vi "ELVIS III v1.0 Coerce AI Scaling.vi"(5 "Max Value":dbl[](array[numeric]), 7 "Min Value":dbl[](array[numeric]), 8 "error in (no error)":errorcluster, 10 "Channel List Size":i32) -> (0 "error out":errorcluster, 2 "Scale Constants Array":T1)   [LabVIEW 2021]
uses:
  <vilib>/myRIO/Common/Instrument Driver Framework/Utilities/typedefs/Analog Scaling Constants List.ctl
  <vilib>/myRIO/Common/Instrument Driver Framework/Utilities/typedefs/Analog Scaling Constants.ctl
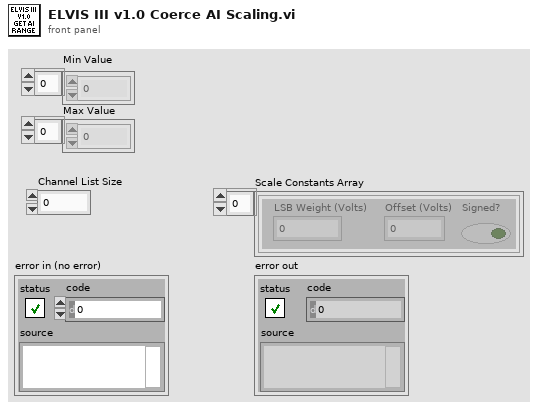
[diagram p1: front panel]
types:
  T1 = typedef "Analog Scaling Constants List.ctl" = T2[]
  T2 = typedef "Analog Scaling Constants.ctl" = cluster{"LSB Weight (Volts)":dbl, "Offset (Volts)":dbl, "Signed?":bool}
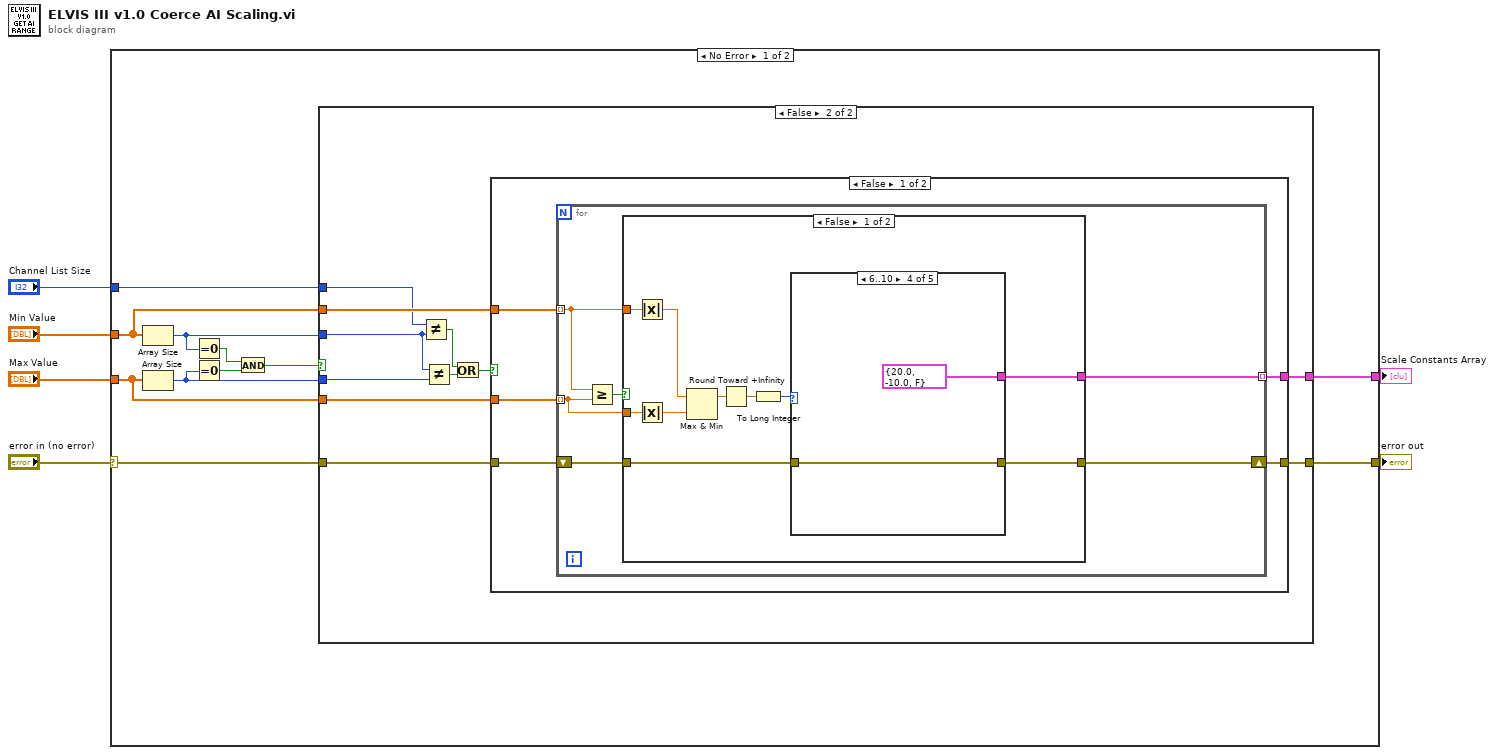
[diagram p0: block diagram]
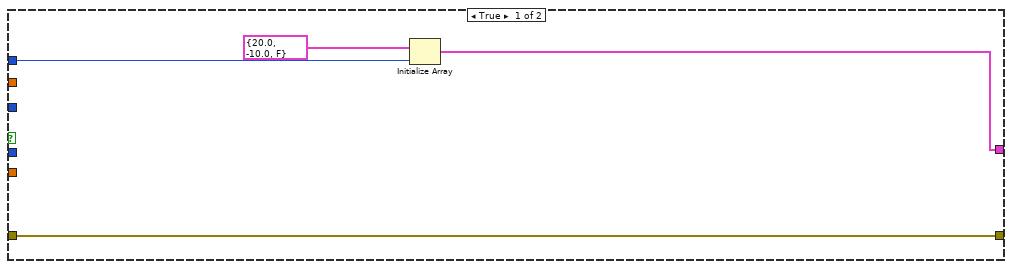
[diagram p2: hidden frame]
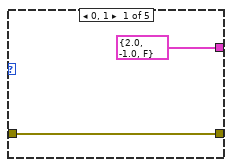
[diagram p3: hidden frame]
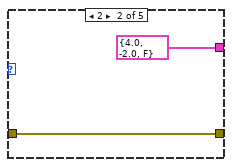
[diagram p4: hidden frame]
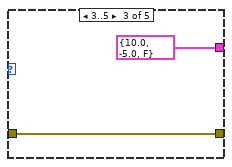
[diagram p5: hidden frame]
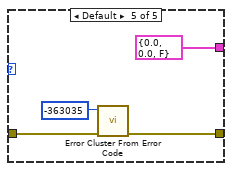
[diagram p6: hidden frame]
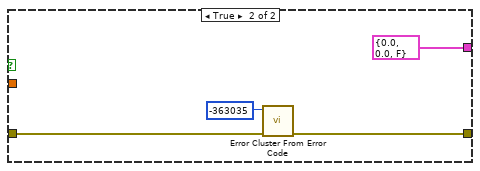
[diagram p7: hidden frame]
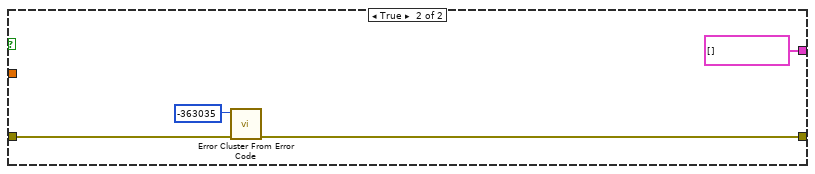
[diagram p8: hidden frame]
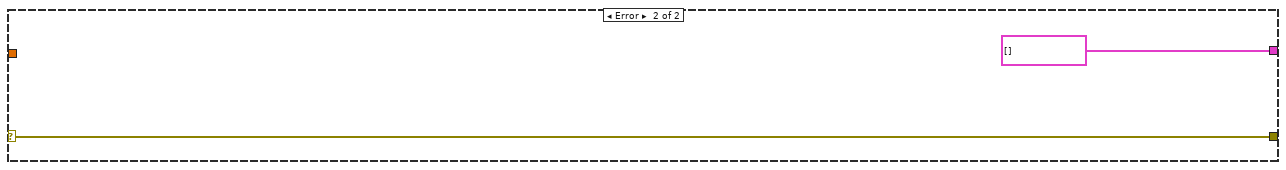
[diagram p9: hidden frame]
diagram:
  n1 = case shown="No Error" "error in (no error)" {
    selector: "error in (no error)" -> [w17 w75]
    tunnel: [w16 w75] -> w5
    tunnel: "Min Value" -> [w15 _]
    tunnel: "Max Value" -> [w14 _]
    tunnel: [w13 T2[] []] -> w2
    tunnel: "Channel List Size" -> [w12 _]
    frame No Error {
      n2 = Array Size(array=w15) -> (size(s)=w11:i32)
      n3 = Array Size(array=w14) -> (size(s)=w10:i32)
      n4 = Equal To 0?(x=w11) -> (x = 0?=w9:bool)
      n5 = Equal To 0?(x=w10) -> (x = 0?=w8:bool)
      n6 = And(x=w9, y=w8) -> (x .and. y?=w7:bool)
      n7 = case shown="False" w7 {
        tunnel: w17 -> [w21 w29]
        tunnel: [w21 w28] -> w16
        tunnel: w15 -> [_ w27]
        tunnel: w14 -> [_ w26]
        tunnel: [w18 w25] -> w13
        tunnel: w12 -> [w19 w24]
        tunnel: w11 -> [_ w23]
        tunnel: w10 -> [_ w22]
        frame True {
          n8 = Initialize Array(T2 {"LSB Weight (Volts)"=20.0, "Offset (Volts)"=-10.0, "Signed?"=FALSE} ("output cluster"), w19) -> (w18:T2[])
        }
        frame False {
          n9 = Not Equal?(x=w24, y=w23) -> (x != y?=w32:bool)
          n10 = Not Equal?(x=w23, y=w22) -> (x != y?=w31:bool)
          n11 = Or(x=w32, y=w31) -> (x .or. y?=w30:bool)
          n12 = case shown="False" w30 {
            tunnel: w29 -> [w35 w72]
            tunnel: [w34 w71] -> w28
            tunnel: w27 -> [w37 _]
            tunnel: w26 -> [w36 _]
            tunnel: [w33 T2[] []] -> w25
            frame False {
              n13 = for {
                tunnel: w37 -> [w40] mode=indexing
                tunnel: w36 -> [w39] mode=indexing
                shift-right: [w41] -> w34
                shift-left: w35 -> [w42]
                tunnel: [w38] -> w33 mode=indexing
                n14 = Greater Or Equal?(x=w40, y=w39) -> (x >= y?=w43:bool)
                n15 = case shown="False" w43 {
                  tunnel: w42 -> [w45 w68]
                  tunnel: [w44 w67] -> w41
                  tunnel: w40 -> [w53 _]
                  tunnel: w39 -> [w52 _]
                  tunnel: [w46 T2 {"LSB Weight (Volts)"=0.0, "Offset (Volts)"=0.0, "Signed?"=FALSE} ("Analog Scaling Constants")] -> w38
                  frame False {
                    n16 = Absolute Value(x=w53) -> (abs(x)=w51:dbl)
                    n17 = Absolute Value(x=w52) -> (abs(x)=w50:dbl)
                    n18 = Max & Min(x=w51, y=w50) -> (max(x,y)=w48:dbl)  [unwired: 1 out]
                    n19 = Round Toward +Infinity(x=w48) -> (ceil(x): smallest int >= x=w47:dbl)
                    n20 = To Long Integer(number=w47) -> (32bit integer=w49:i32)
                    n21 = case shown="6..10" w49 {
                      tunnel: [T2 {"LSB Weight (Volts)"=2.0, "Offset (Volts)"=-1.0, "Signed?"=FALSE} ("output cluster") T2 {"LSB Weight (Volts)"=4.0, "Offset (Volts)"=-2.0, "Signed?"=FALSE} ("output cluster") T2 {"LSB Weight (Volts)"=10.0, "Offset (Volts)"=-5.0, "Signed?"=FALSE} ("output cluster") T2 {"LSB Weight (Volts)"=20.0, "Offset (Volts)"=-10.0, "Signed?"=FALSE} ("output cluster") T2 {"LSB Weight (Volts)"=0.0, "Offset (Volts)"=0.0, "Signed?"=FALSE} ("output cluster")] -> w46
                      tunnel: w45 -> [w54 w56 w58 w60 w64]
                      tunnel: [w54 w56 w58 w60 w63] -> w44
                      frame 0, 1 {
                      }
                      frame 2 {
                      }
                      frame 3..5 {
                      }
                      frame 6..10 {
                      }
                      frame Default {
                        n22 = call <vilib>:"Error Cluster From Error Code.vi"("error in (no error)"=w64, "error code (0)"=-363035) -> ("error out"=w63:errorcluster)  [unwired: 7 in]
                      }
                    }
                  }
                  frame True {
                    n23 = call <vilib>:"Error Cluster From Error Code.vi"("error in (no error)"=w68, "error code (0)"=-363035) -> ("error out"=w67:errorcluster)  [unwired: 7 in]
                  }
                }
              }
            }
            frame True {
              n24 = call <vilib>:"Error Cluster From Error Code.vi"("error in (no error)"=w72, "error code (0)"=-363035) -> ("error out"=w71:errorcluster)  [unwired: 7 in]
            }
          }
        }
      }
    }
    frame Error {
    }
  }
  "error out" <- w5
  "Scale Constants Array" <- w2
